vi "string.vi"() -> ()   [LabVIEW 2020]
panel:
  out "date/time string":string
  out "resulting string":string
  out "output 1":dbl
  out "after substring":string
  out "match substring":string
  out "before substring":string
  out "result string":string
  out "substring":string
  out "concatenated string":string
  out "length":i32
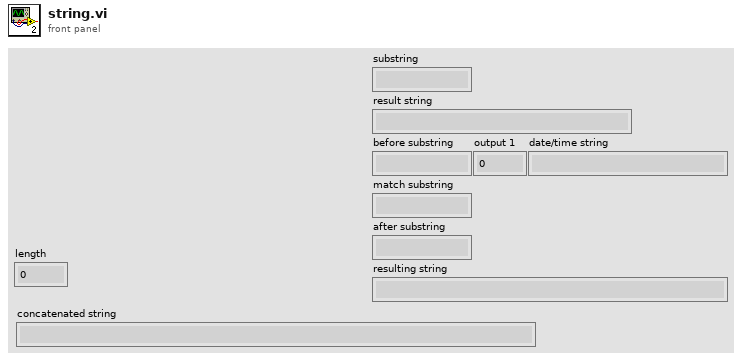
[diagram p1: front panel]
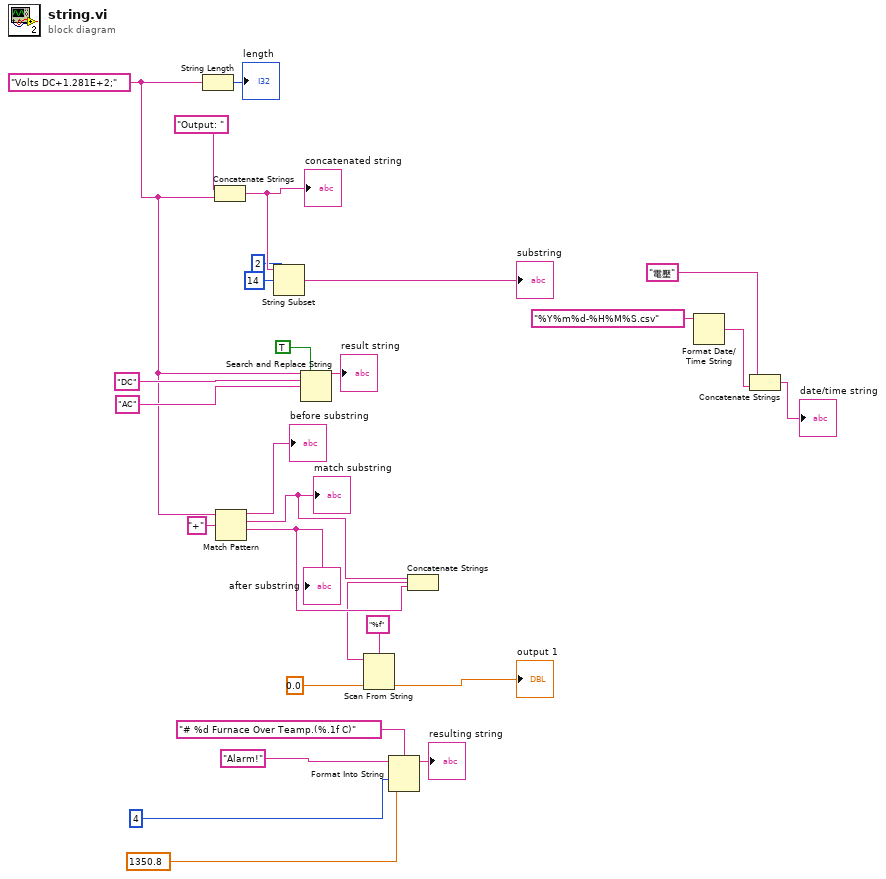
[diagram p0: block diagram]
diagram:
  w18 = "Volts DC+1.281E+2;"
  n1 = String Length(string=w18) -> (length=→"length":i32)
  n2 = Concatenate Strings("Output: " ("string"), w18) -> (w26:string)
  "concatenated string" <- w26
  n3 = Match Pattern(string=w18, regular expression="+") -> (before substring=→"before substring":string, match substring=w15:string, after substring=w14:string)  [unwired: 1 in, 1 out]
  "match substring" <- w15
  "after substring" <- w14
  n4 = String Subset(string=w26, offset (0)=14, length (rest)=2 ("length (rest)")) -> (substring=→"substring":string)
  n5 = Search and Replace String(replace all?=TRUE ("replace all? (F)"), input string=w18, search string="DC", replace string="AC" ("replace string (\"\")")) -> (result string=→"result string":string)  [unwired: 4 in, 3 out]
  n6 = Format Into String(format string="# %d Furnace Over Teamp.(%.1f C)", initial string="Alarm!", 4, 1350.8) -> (resulting string=→"resulting string":string)  [unwired: 1 in, 1 out]
  n7 = Concatenate Strings(w15, w14) -> (w13:string)
  n8 = Scan From String(format string="%f", input string=w13, default 1=0.0) -> (output 1=→"output 1":dbl)  [unwired: 2 in, 3 out]
  n9 = Format Date/Time String(time format string (%c)="%Y%m%d-%H%M%S.csv") -> (date/time string=w3:string)  [unwired: 2 in]
  n10 = Concatenate Strings("電壓", w3) -> (→"date/time string":string)
